vi "isConnected.vi"(8 "error in (no error)":errorcluster, 11 "AlCS in":refnum<class "AlCS.lvclass">) -> (0 "error out":errorcluster, 2 "conneced?":bool, 3 "AlCS out":refnum<class "AlCS.lvclass">)   [LabVIEW 2016, in "AlCS.lvclass"]
uses:
  AlCS.lvclass
  AlCS.lvclass/AlCS.ctl
  ts_labview_tcp/TCPClient/TCPClient.lvclass
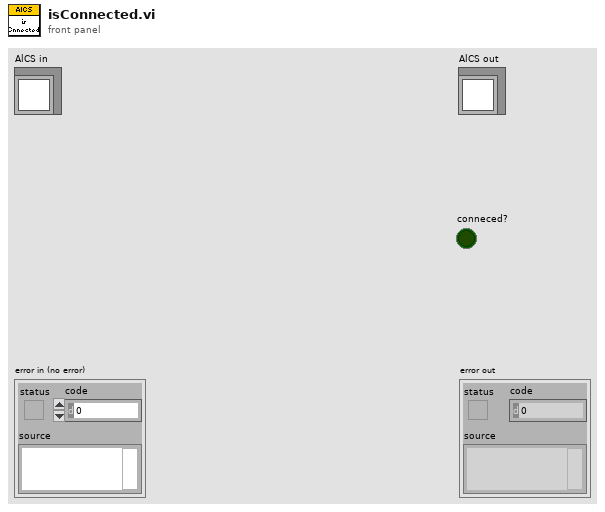
[diagram p1: front panel]
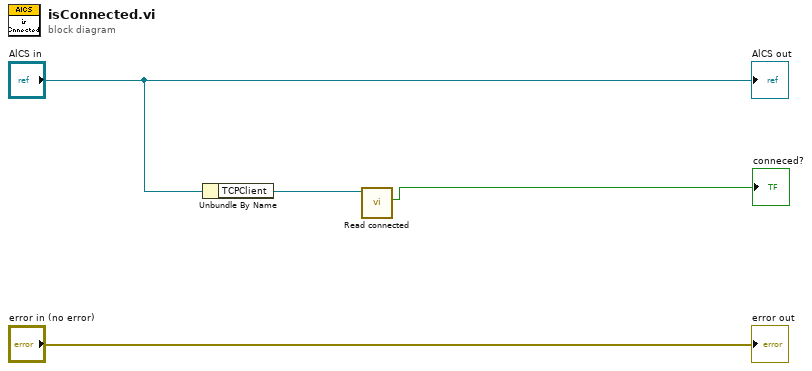
[diagram p0: block diagram]
diagram:
  n1 = Unbundle By Name("AlCS in") -> ("TCPClient"=w2:refnum<class "TCPClient.lvclass">)
  n2 = call-dynamic "Read connected.vi"("TCPCommunicator in"=w2) -> ("connected"=→"conneced?":bool)  [unwired: 8 in, 2 out]
  "error out" <- "error in (no error)"
  "AlCS out" <- "AlCS in"
